vi "cv_potential_waveform.vi"() -> ()   [LabVIEW 2019]
panel:
  out "# of collisions":i32
  out "VTrack":dbl(graph)
  in  "stop":bool
  in  "PositiveScan?":bool
  in  "cycle":i32
  in  "Vstep V/step":dbl format="%#_13g"
  in  "Scanrate V/s":dbl format="%#_13g"
  in  "LowV":dbl format="%#_13g"
  in  "HighV":dbl format="%#_13g"
  in  "InitV":dbl format="%#_13g"
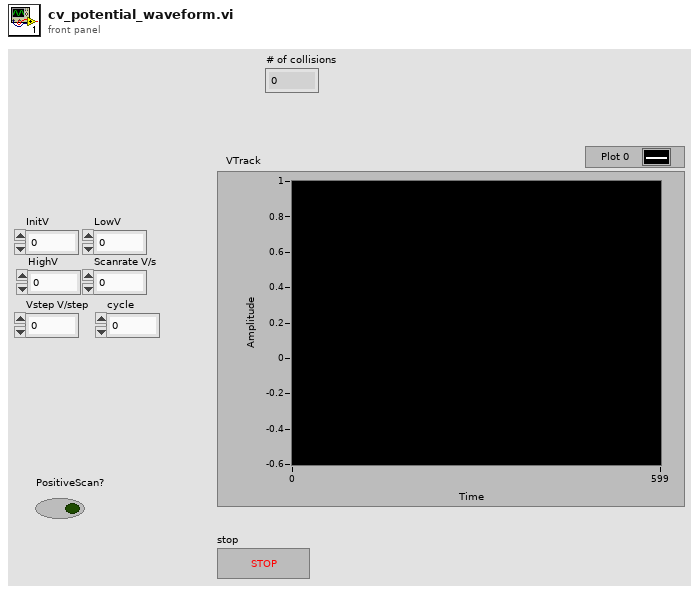
[diagram p1: front panel]
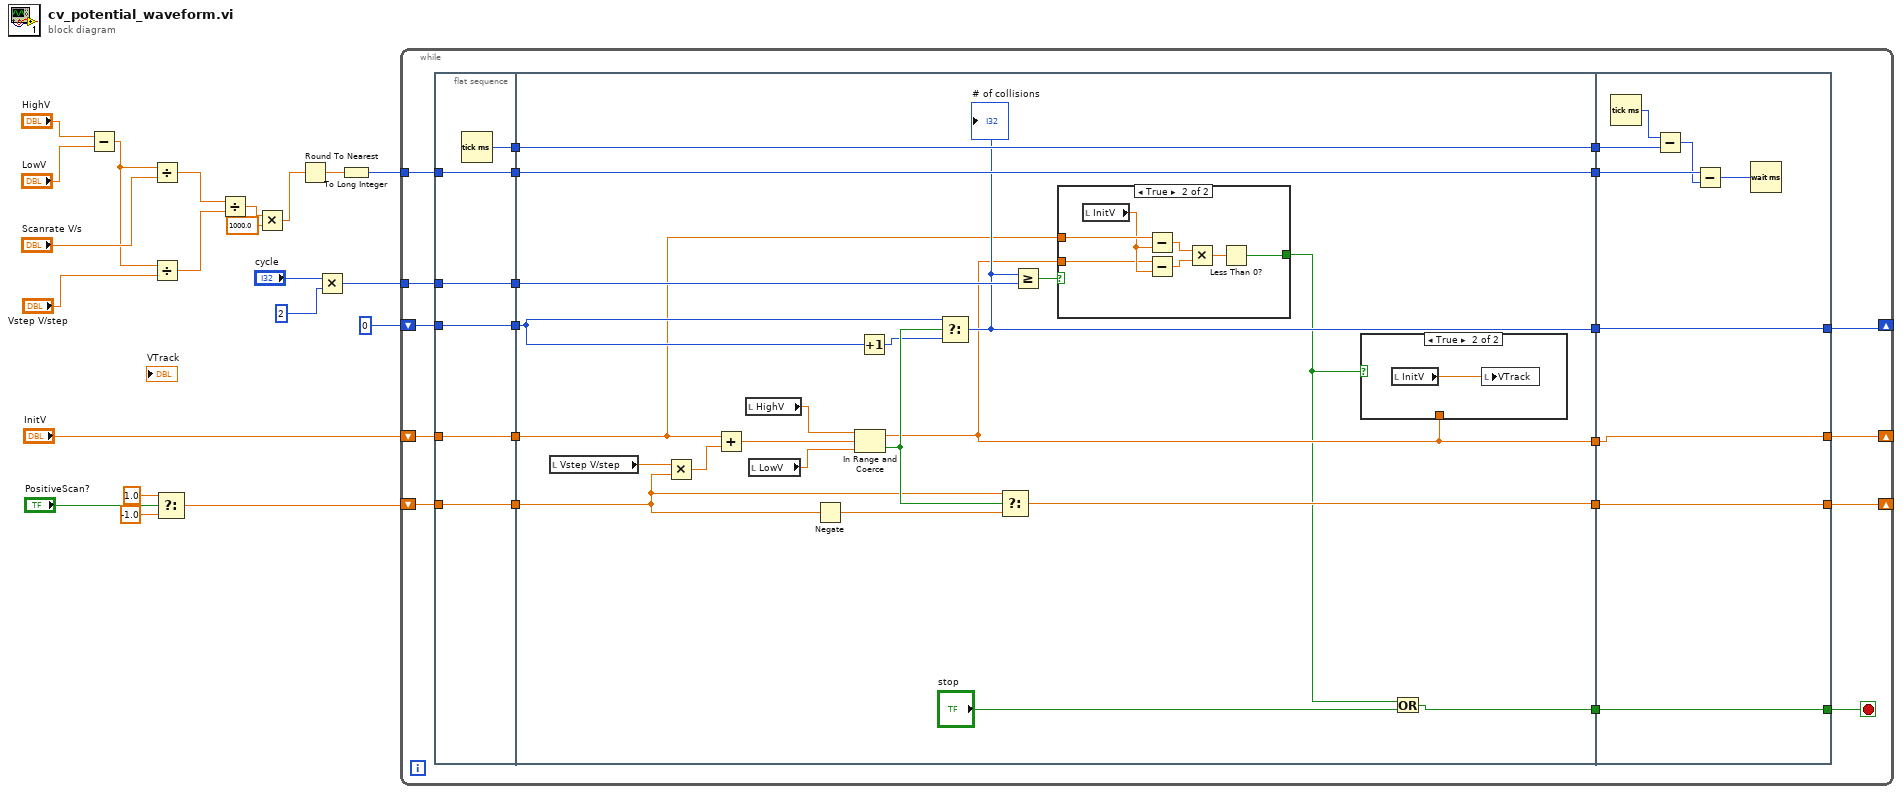
[diagram p0: block diagram]
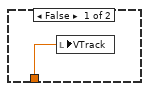
[diagram p2: hidden frame]
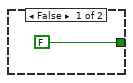
[diagram p3: hidden frame]
diagram:
  n1 = Subtract(x="HighV", y="LowV") -> (x-y=w1:dbl)
  n2 = Divide(x=w1, y="Scanrate V/s") -> (x/y=w13:dbl)
  n3 = Divide(x=w1, y="Vstep V/step") -> (x/y=w12:dbl)
  n4 = Select(t=1.0, s="PositiveScan?", f=-1.0) -> (s? t:f=w6:dbl)
  n5 = Divide(x=w13, y=w12) -> (x/y=w9:dbl)
  n6 = Multiply(x=w9, y=1000.0) -> (x*y=w7:dbl)
  n7 = Round To Nearest(number=w7) -> (nearest integer value=w11:dbl)
  n8 = Multiply(x="cycle", y=2) -> (x*y=w2:i32)
  n9 = To Long Integer(number=w11) -> (32bit integer=w10:i32)
  n10 = while {
    shift-right: [w32] -> _
    shift-left: "InitV" -> [w36]
    tunnel: w10 -> [w42]
    shift-right: [w30] -> _
    shift-left: w6 -> [w34]
    shift-right: [w26] -> _
    shift-left: 0 -> [w28]
    tunnel: w2 -> [w22]
    stop <- w24 stop-if-true
    n11 = flat-sequence {
      tunnel: w42 -> [w47]
      tunnel: [w48] -> w41
      tunnel: [w47] -> w39
      tunnel: [w46] -> w37
      tunnel: w36 -> [w46]
      tunnel: [w45] -> w35
      tunnel: w34 -> [w45]
      tunnel: [w44] -> w29
      tunnel: w28 -> [w44]
      tunnel: [w43] -> w23
      tunnel: w22 -> [w43]
      tunnel: w41 -> [w69]
      tunnel: [w69] -> w40
      tunnel: w39 -> [w68]
      tunnel: [w68] -> w38
      tunnel: w37 -> [w52]
      tunnel: w35 -> [w55]
      tunnel: [w53] -> w33
      tunnel: [w61] -> w31
      tunnel: w29 -> [w59]
      tunnel: [w56] -> w27
      tunnel: [w50] -> w25
      tunnel: w23 -> [w57]
      tunnel: w40 -> [w87]
      tunnel: w38 -> [w86]
      tunnel: w33 -> [w83]
      tunnel: [w83] -> w32
      tunnel: w31 -> [w82]
      tunnel: [w82] -> w30
      tunnel: w27 -> [w81]
      tunnel: [w81] -> w26
      tunnel: [w80] -> w24
      tunnel: w25 -> [w80]
      frame #0 {
        n12 = Tick Count (ms)() -> (millisecond timer value=w48:u32)
      }
      frame #1 {
        n13 = local read "Vstep V/step"() -> (w67:dbl)
        n14 = Multiply(x=w67, y=w55) -> (x*y=w66:dbl)
        n15 = Add(x=w52, y=w66) -> (x+y=w65:dbl)
        n16 = local read "HighV"() -> (w63:dbl)
        n17 = local read "LowV"() -> (w64:dbl)
        n18 = Negate(x=w55) -> (-x=w62:dbl)
        n19 = In Range and Coerce(upper limit=w63, x=w65, lower limit=w64) -> (coerced(x)=w53:dbl, In Range?=w60:bool)
        n20 = Increment(x=w59) -> (x+1=w58:i32)
        n21 = Select(t=w59, s=w60, f=w58) -> (s? t:f=w56:i32)
        "# of collisions" <- w56
        n22 = Select(t=w55, s=w60, f=w62) -> (s? t:f=w61:dbl)
        n23 = Greater Or Equal?(x=w56, y=w57) -> (x >= y?=w54:bool)
        n24 = case shown="True" w54 {
          tunnel: w53 -> [_ w77]
          tunnel: w52 -> [_ w79]
          tunnel: [FALSE w73] -> w49
          frame False {
          }
          frame True {
            n25 = local read "InitV"() -> (w78:dbl)
            n26 = Subtract(x=w79, y=w78) -> (x-y=w76:dbl)
            n27 = Subtract(x=w77, y=w78) -> (x-y=w75:dbl)
            n28 = Multiply(x=w76, y=w75) -> (x*y=w74:dbl)
            n29 = Less Than 0?(x=w74) -> (x < 0?=w73:bool)
          }
        }
        n30 = case shown="True" w49 {
          tunnel: w53 -> [w70 _]
          frame False {
            n31 = local write "VTrack"(w70) -> ()
          }
          frame True {
            n32 = local read "InitV"() -> (w71:dbl)
            n33 = local write "VTrack"(w71) -> ()
          }
        }
        n34 = Or(x=w49, y="stop") -> (x .or. y?=w50:bool)
      }
      frame #2 {
        n35 = Tick Count (ms)() -> (millisecond timer value=w88:u32)
        n36 = Subtract(x=w88, y=w87) -> (x-y=w85:u32)
        n37 = Subtract(x=w86, y=w85) -> (x-y=w84:u32)
        n38 = Wait (ms)(milliseconds to wait=w84) -> ()  [unwired: 1 out]
      }
    }
  }
